vi "Config Test.vi"(8 "Error In":errorcluster, 10 "Debug":bool, 11 "Station":T1(ring)) -> (0 "Error Out":errorcluster)   [LabVIEW 2019, in "Unit Test Engine Tools.lvlib"]
uses:
  Unit Test Engine Tools.lvlib
  d678025b-0795-4d1f-a448-38ac89b15b22.vi
  LVUT Global 1.vi
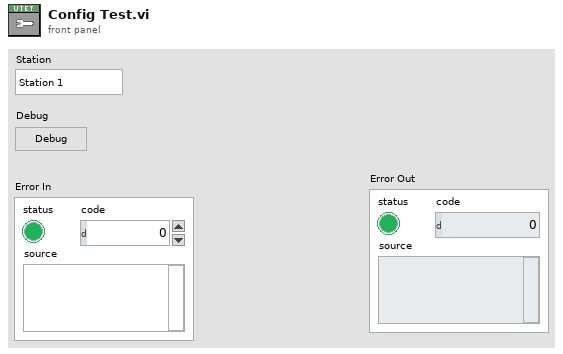
[diagram p1: front panel]
types:
  T1 = enum16{"Station 1", "Station 2", "Station 3", "Station 4"}
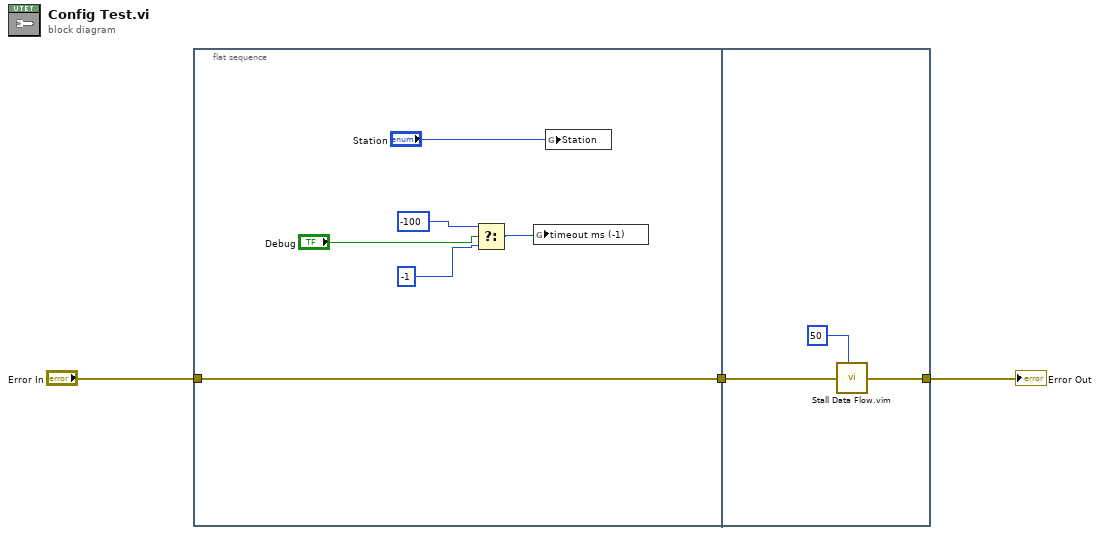
[diagram p0: block diagram]
diagram:
  n1 = flat-sequence {
    tunnel: "Error In" -> [w4]
    tunnel: [w4] -> w2
    tunnel: [w11] -> w1
    tunnel: w2 -> [w12]
    frame #0 {
      n2 = Select(t=-100, s="Debug", f=-1 ("timeout ms (-1)")) -> (s? t:f=w5:i32)
      n3 = global write "LVUT Global 1.vi" "timeout ms (-1)"(w5) -> ()
      n4 = global write "LVUT Global 1.vi" "Station"("Station") -> ()
    }
    frame #1 {
      n5 = call "Stall Data Flow.vim"("value in"=w12, "milliseconds to wait"=u32 50) -> ("value out"=w11:errorcluster)  [unwired: 1 out]
    }
  }
  "Error Out" <- w1
